vi "Initialize first data (Record).vi"(1 "Оператор":string, 2 "Получаемый материал":string) -> (0 "Выходные данные":string)   [LabVIEW 2016]
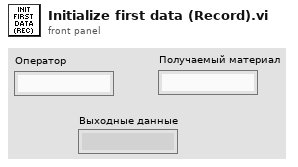
[diagram p1: front panel]
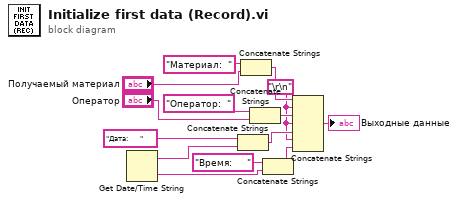
[diagram p0: block diagram]
diagram:
  w4 = "\r\n"
  n1 = Get Date/Time String() -> (date string=w10:string, time string=w9:string)  [unwired: 3 in]
  n2 = Concatenate Strings("Дата:      " ("string"), w10) -> (w13:string)
  n3 = Concatenate Strings("Материал:  " ("string"), "Получаемый материал") -> (w5:string)
  n4 = Concatenate Strings("Оператор:  " ("string"), "Оператор") -> (w14:string)
  n5 = Concatenate Strings("Время:     " ("string"), w9) -> (w12:string)
  n6 = Concatenate Strings(w5, w4, w14, w4, w13, w4, w12) -> (→"Выходные данные":string)
